vi "Create Filter from Zero-Pole-Gain.vi"() -> ()   [LabVIEW 2023]
doc: "Demonstrates how to use the DFD Build Filter from Zero-Pole-Gain VI to create a filter from the zeroes, poles, and gain.\n\nComplete the following steps to use this VI.\n1) Run the VI.\n2) Add a zero or pole.\n3) Observe the Z-Plane graph to see the zero or pole appear at the expected position.\n4) Delete a zero or pole.\n5) Observe the Z-Plane graph to see the zero or pole disappear at the expected position.\n\n<B>Note:</B> The complex zeroes/poles must appear in conjugate pairs. Otherwise, the resulting zeroes/poles might be different from what you expect."
uses:
  <vilib>/addons/Digital Filter Design/_Objects.llb/DFD Pole-Zero Plot.ctl
  <vilib>/addons/Digital Filter Design/NI_DigFilterLicensed.lvlib
panel:
  out "Error Message":string
  in  "Gain":dbl=1.0 format="%.2f"
  in  "Poles":cdb[](array[numeric])=[0.8+0.0i] format="%.2f"
  in  "Zeroes":cdb[](array[numeric])=[0.3+0.4i, 0.3-0.4i, 1.2+1.6i, 1.2-1.6i, 1.0+0.0i] format="%.2f"
  out "Z-Plane":T1
  # "Select Help>>Show Context Help and move the cursor over the VI icon for more information."
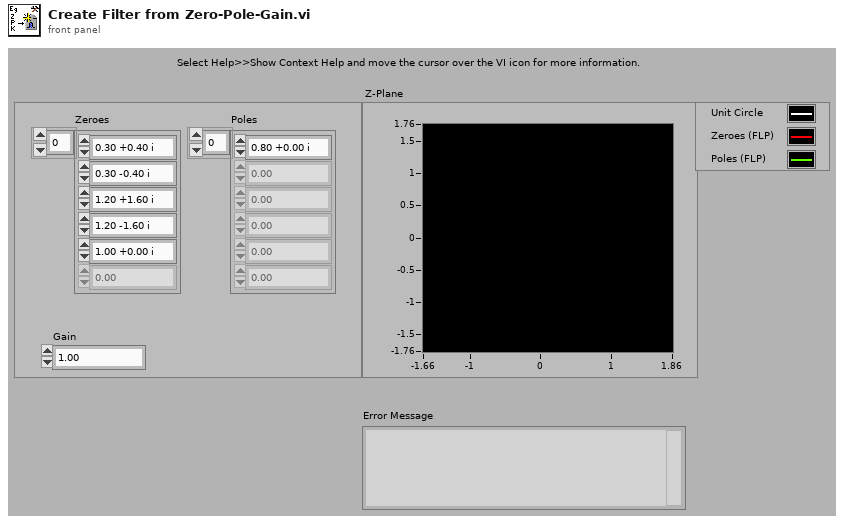
[diagram p1: front panel]
types:
  T1 = typedef "NI_DigFilterLicensed.lvlib/DFD Pole-Zero Plot.ctl" = cluster{dbl[], dbl[]}[]
  T2 = typedef "NI_DigFilterLicensed.lvlib/DFD Filter Obj.ctl" = cluster{"mSRate_Fs":dbl, "mSRate_Version":string, "mSRate_Comments":string, "mSRate_OrgCoef":T3, "mSRate_CurCoef":T3, "mSRate_Quantized?":bool, "mSRate_QCoef":T3, "mSRate_QSettings":T5[], "mSRate_Order":i32, "mSRate_Scaling":cluster{"mSRate_ScaleByPowerOf2?":bool, "mSRate_ScaleType":T7}}
  T3 = typedef "NI_DigFilterLicensed.lvlib/DFD Filter Coef.ctl" = cluster{"type":T4, "gain":dbl, "coef a (k)":dbl[], "coef b (v)":dbl[]}
  T4 = typedef "NI_DigFilterLicensed.lvlib/DFD Filter Structure Type Selector.ctl" = enum16{"Undefined", "FIR Direct Form", "FIR Direct Form Transposed", "FIR Symmetric", "FIR Antisymmetric", "IIR Direct Form I", "IIR Direct Form I Transposed", "IIR Direct Form II", "IIR Direct Form II Transposed", "IIR Cascaded Second Order Sections Form I", "IIR Cascaded Second Order Sections Form I Transposed", "IIR Cascaded Second Order Sections Form II", "IIR Cascaded Second Order Sections Form II Transposed", "Lattice Allpass (basic sections)", "Lattice Allpass (one multiplier sections)", "Lattice Allpass (normalized sections)", "Lattice AR (basic sections)", "Lattice AR (one multiplier sections)", "Lattice AR (normalized sections)", "Lattice MA (minimum phase)", "Lattice MA (maximum phase)", "Lattice ARMA (basic sections)", "Lattice ARMA (one multiplier sections)", "Lattice ARMA (normalized sections)"}
  T5 = typedef "NI_DigFilterLicensed.lvlib/dfd_Internal Quantization Settings.ctl" = cluster{"source":T6, "wl":i16, "iwl":i16, "overflow mode":enum16{"Saturation", "Wrap"}, "rounding mode":enum16{"Nearest", "Truncation"}, "signed?":bool}
  T6 = typedef "NI_DigFilterLicensed.lvlib/dfd_Internal Quantization Srcs.ctl" = u16
  T7 = typedef "NI_DigFilterLicensed.lvlib/DFD Coef Norm Type.ctl" = enum16{"No Norm", "Time Domain 1-Norm", "Time Domain 2-Norm", "Time Domain Inf-Norm"}
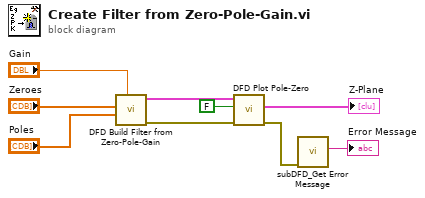
[diagram p0: block diagram]
diagram:
  n1 = call <vilib>:"DFD Build Filter from Zero-Pole-Gain.vi"("gain"="Gain", "poles"="Poles", "zeroes"="Zeroes") -> ("error out"=w8:errorcluster, "filter out"=w9:T2)  [unwired: 2 in, 5 out]
  n2 = call <vilib>:"DFD Plot Pole-Zero.vi"("error in (no error)"=w8, "upper half plane only"=FALSE, "filter in"=w9) -> ("error out"=w1:errorcluster, "Z-Plane"=→"Z-Plane":T1)  [unwired: 7 out]
  n3 = call <vilib>:"subDFD_Get Error Message.vi"("error in (no error)"=w1) -> ("Error Message"=→"Error Message":string)  [unwired: 10 out]
